vi "Configure Multi Eval Meas List Segment SEM.vi"(4 "SEM Enable (Off)":bool, 5 "OBW Enable (Off)":bool, 6 "Enable (Off)":bool, 7 "Statistics (20)":i32=20, 8 "error in (no error)":errorcluster, 9 "Segment (1)":i32=1, 10 "Instance (1)":T1=1, 11 "VISA resource name":refnum<visa-resource-name>) -> (0 "error out":errorcluster, 3 "VISA resource name out":refnum<visa-resource-name>)   [LabVIEW 2020, in "Rohde&Schwarz CMWXP NR FR1 Measurement.lvlib"]
doc: "Defines settings for spectrum emission measurements in list mode for segment <no>.\n\nAttribute:\nRSCMWXPNRFR1M_ATTR_MULTI_EVAL_MEAS_LIST_SEGMENT_SEM\n\nRemote-control command:\nCONFigure:NRSub:MEAS<i>:MEValuation:LIST:SEGMent<no>:SEMask"
uses:
  <instrlib>/Rohde&Schwarz CMWXP NR FR1 Measurement/Rohde&Schwarz CMWXP NR FR1 Measurement.lvlib
  <instrlib>/Rohde&Schwarz CMWXP NR FR1 Measurement/Private/_Instance.ctl
  <instrlib>/Rohde&Schwarz CMWXP NR FR1 Measurement/Private/rsidr_core.llb/rsidr_core.lvlib
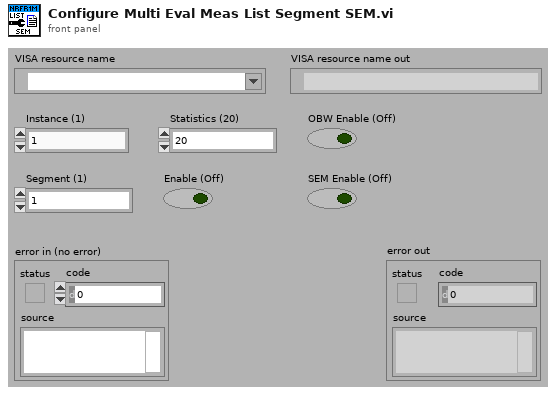
[diagram p1: front panel]
types:
  T1 = typedef "Rohde&Schwarz CMWXP NR FR1 Measurement.lvlib/_Instance.ctl" = i32
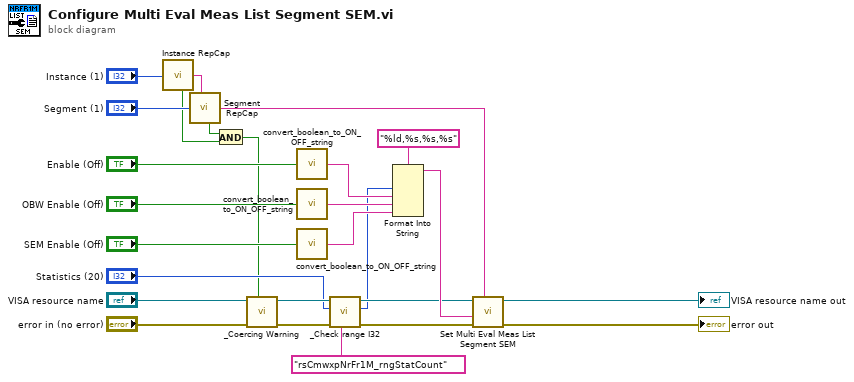
[diagram p0: block diagram]
diagram:
  n1 = call <instrlib>:"Instance RepCap.vi"("Instance In"="Instance (1)") -> ("In Range?"=w3:bool, "RepCap Identifier Out"=w22:string)  [unwired: 1 in]
  n2 = call <instrlib>:"Segment RepCap.vi"("Segment In"="Segment (1)", "RepCap String In (\"\")"=w22) -> ("In Range?"=w2:bool, "RepCap Identifier Out"=w21:string)
  n3 = And(x=w2, y=w3) -> (x .and. y?=w1:bool)
  n4 = call <instrlib>:"_Coercing Warning.vi"("In Range?"=w1, "error in (no error)"="error in (no error)", "VISA resource name"="VISA resource name") -> ("error out"=w9:errorcluster, "VISA resource name out"=w8:refnum<visa-resource-name>)  [unwired: 7 in]
  n5 = call <instrlib>:"convert_boolean_to_ON_OFF_string.vi"("boolean value in"="Enable (Off)") -> ("string value out"=w15:string)  [unwired: 4 in]
  n6 = call <instrlib>:"convert_boolean_to_ON_OFF_string.vi"("boolean value in"="OBW Enable (Off)") -> ("string value out"=w14:string)  [unwired: 4 in]
  n7 = call <instrlib>:"convert_boolean_to_ON_OFF_string.vi"("boolean value in"="SEM Enable (Off)") -> ("string value out"=w13:string)  [unwired: 4 in]
  n8 = call <instrlib>:"_Check range I32.vi"("Range Table Identifier"="rsCmwxpNrFr1M_rngStatCount", "error in (no error)"=w9, "I32 Value In"="Statistics (20)", "VISA resource name"=w8) -> ("error out"=w7:errorcluster, "I32 Value Out"=w4:i32, "VISA resource name out"=w6:refnum<visa-resource-name>)  [unwired: 5 in]
  n9 = Format Into String(format string="%ld,%s,%s,%s", w4, w15, w14, w13) -> (resulting string=w19:string)  [unwired: 2 in, 1 out]
  n10 = call "Set Multi Eval Meas List Segment SEM"("Repeated Capabilities"=w21, "error in (no error)"=w7, "Multi Eval Meas List Segment SEM ()"=w19, "instrument handle"=w6) -> ("error out"=→"error out":errorcluster, "instrument handle out"=→"VISA resource name out":refnum<visa-resource-name>)  [unwired: 6 in]
